vi "LOG Save.vi"(8 "error in (no error)":errorcluster, 10 "Message Data":variant, 11 "Data Cluster":T1) -> (0 "error out":errorcluster, 3 "Data Cluster out":T1)   [LabVIEW 2020, in "LOG.lvlib"]
uses:
  LOG.lvlib
  LOG Configuration.ctl
  support/Message Queue/Message Cluster.ctl
  <vilib>/Utility/file.llb/Write Delimited Spreadsheet (string).vi
  support/Message Queue/Message Queue.lvlib
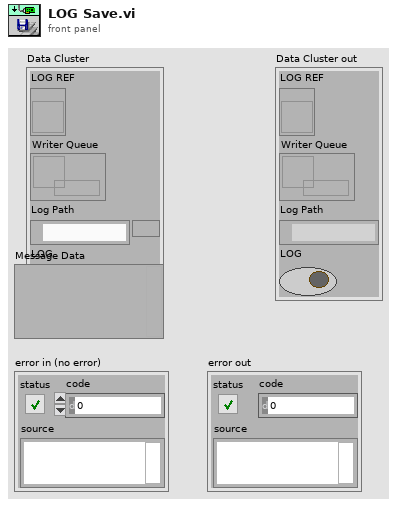
[diagram p1: front panel]
types:
  T1 = typedef "LOG.lvlib/LOG Configuration.ctl" = cluster{"LOG REF":refnum<vi>, "Writer Queue":refnum<queue>, "Log Path":path, "LOG":bool}
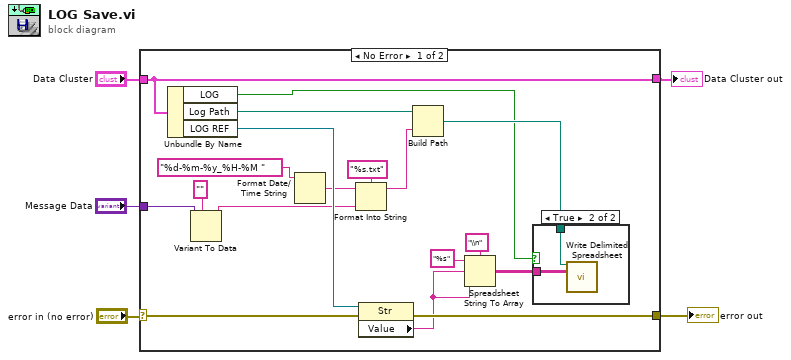
[diagram p0: block diagram]
diagram:
  n1 = case shown="No Error" "error in (no error)" {
    selector: "error in (no error)" -> [w21 w26]
    tunnel: [w7 w27] -> w4
    tunnel: "Data Cluster" -> [w7 w27]
    tunnel: [w23 w26] -> w3
    tunnel: "Message Data" -> [w20 _]
    frame No Error {
      n2 = Unbundle By Name(w7) -> ("LOG"=w6:bool, "Log Path"=w14:path, "LOG REF"=w22:refnum<vi>)
      n3 = Variant To Data(type="" ("delimiter (Tab)"), Variant=w20) -> (data=w10:string)  [unwired: 1 in, 1 out]
      n4 = Format Date/Time String(time format string (%c)="%d-%m-%y_%H-%M ") -> (date/time string=w12:string)  [unwired: 2 in]
      n5 = Format Into String(format string="%s.txt", initial string=w12, w10) -> (resulting string=w9:string)  [unwired: 1 in, 1 out]
      n6 = property class="Str"(reference=w22, error in=w21) -> (error out=w23:errorcluster, "Value"=w19:string)  [unwired: 1 out]
      n7 = Build Path(base path=w14, name or relative path=w9) -> (appended path=w8:path)
      n8 = Spreadsheet String To Array(delimiter (Tab)="\\n", format string="%s", spreadsheet string=w19, array type (2D Dbl)=w19) -> (array=w18:string[][])
      n9 = case shown="True" w6 {
        tunnel: w18 -> [_ w24]
        tunnel: w8 -> [_ w25]
        frame False {
        }
        frame True {
          n10 = call-poly <vilib>:"Write Delimited Spreadsheet.vi"("file path (dialog if empty)"=w25, "2D data"=w24) -> ()  [unwired: 12 in, 2 out]
        }
      }
    }
    frame Error {
    }
  }
  "error out" <- w3
  "Data Cluster out" <- w4
